vi "BuildAllFileNames.vi"(8 "Reset?":bool, 11 "Settings":T1={"Name of test"="", "Date"=timestamp(0 s since 1904-01-01), "Location"="", "Template"="", "Soundcard"="", "resolution"=32, "Sampling rate"=48000, "Ch1 Gain "=25.0, "Ch2 Gain"=10.0, "Sample time (s)"=0.3, "Pre-trigger (s)"=0.01, "Hammer Threshold"=10.0, "Positions"=12, "Taps/Position"=5, "Set Names"="", "Freq resolution"=10.0, "Hammer cutoff"=0.0, "Mic cutoff"=0.0, "Double bounce "=0.0, "Hammer Cal"=10.0, "dB Offset"=0.0, "Accel Cal"=10.0, "Vibrometer Cal"=0.0, "Mic Cal"=0.0, "Output"=2, "Voltage Cal"=1.0, "Vibrometer Port"="ASRL27::INSTR", "Range"=4, "High Pass"=2, "Bandwidth"=4, "X Range"=[], "Y Range"=[], "dB Spread"=0.0, "Trigger"=0, "Ch_1"=25, "Ch_2"=25, "flip?"=FALSE, "60Hz"=FALSE, "Time offset"=0.0, "Piezo Cal"=1.0, "Default Notes"=""} {"Ch_2" min=1 step=1; "Ch_1" min=1 max=100 step=1; "Trigger" items=["Hammer (force)", "Self-tap", "Spacebar"]; "Bandwidth" items=["1 kHz"=1, "5 kHz"=5, "10 kHz"=10, "25 kHz"=25, "50 kHz"=50, "100 kHz"=100]; "High Pass" items=["Off", "13 Hz", "104 Hz"]; "Range" items=["10 mm/s"=1, "20 mm/s"=2, "50 mm/s"=5, "100 mm/s"=10, "200 mm/s"=20, "500 mm/s"=50, "1 m/s"=100, "2 m/s"=200]; "Output" items=["Accelerometer", "Speed (from acceleration)", "Microphone", "Vibrometer", "Piezo"]; "Voltage Cal" format="%#_13g"; "Ch2 Gain" format="%#_13g"; "Ch1 Gain" format="%#_13g"; "Double bounce" min=0.0; "Mic cutoff" min=0.0 format="%#_4g"; "Hammer cutoff" min=0.0 format="%#_4g"; "Freq resolution" min=0.0; "Pre-trigger (s)" format="%#_13g"; "Date" format="%<%H:%M\n%d/%m/%y>T"; "resolution" items=["16 bit"=16, "24 bit"=24, "32 bit"=32]; "Sampling rate" items=["22050 samp/s"=22050, "44100 samp/s"=44100, "48000 samp/s"=48000]}) -> (2 "Info":cluster{i32, i32, i32}[](array[cluster]), 3 "File Names":string[](array[string]))   [LabVIEW 2022 SP3]
uses:
  PreferencesControl.ctl
panel:
  # "Hz"
  # "dB"
  # "dB"
  # "sec"
  # "sec"
  # "mV/Pa"
  # "mV/m/s2"
  # "mV/mm/s"
  # "V/N"
  # "sec"
  # "sec"
  # "mV/N"
  # "a.u."
  # "a.u."
  # "sec"
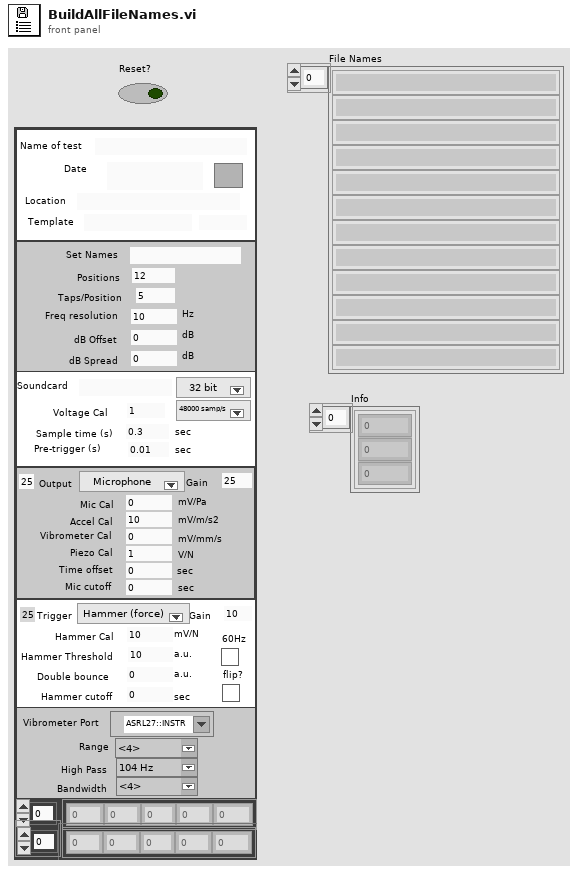
[diagram p1: front panel]
types:
  T1 = typedef "PreferencesControl.ctl" = cluster{"Name of test":string, "Date":timestamp, "Location":string, "Template":string, "Soundcard":string, "resolution":u16, "Sampling rate":u16, "Ch1 Gain ":dbl, "Ch2 Gain":dbl, "Sample time (s)":dbl, "Pre-trigger (s)":dbl, "Hammer Threshold":dbl, "Positions":i16, "Taps/Position":i16, "Set Names":string, "Freq resolution":dbl, "Hammer cutoff":dbl, "Mic cutoff":dbl, "Double bounce ":dbl, "Hammer Cal":dbl, "dB Offset":dbl, "Accel Cal":dbl, "Vibrometer Cal":dbl, "Mic Cal":dbl, "Output":u16, "Voltage Cal":dbl, "Vibrometer Port":refnum<visa-resource-name>, "Range":u16, "High Pass":u16, "Bandwidth":u16, "X Range":cluster{"Minimum":dbl, "Maximum":dbl, "Increment":dbl, "Minor Increment":dbl, "Start":dbl}[], "Y Range":cluster{"Minimum":dbl, "Maximum":dbl, "Increment":dbl, "Minor Increment":dbl, "Start":dbl}[], "dB Spread":dbl, "Trigger":u16, "Ch_1":u8, "Ch_2":u8, "flip?":bool, "60Hz":bool, "Time offset":dbl, "Piezo Cal":dbl, "Default Notes":string}
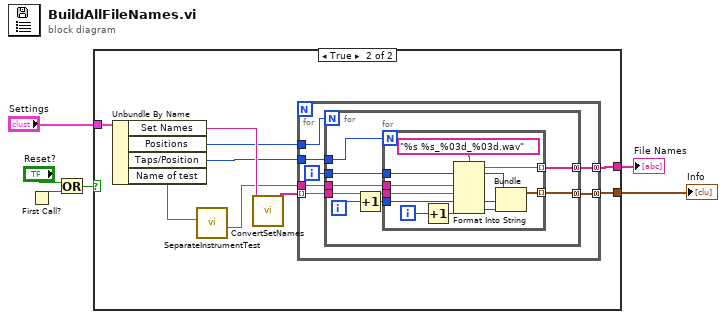
[diagram p0: block diagram]
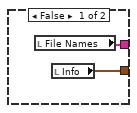
[diagram p2: hidden frame]
diagram:
  n1 = First Call?() -> (First Call?: T/F=w3:bool)
  n2 = Or(x="Reset?", y=w3) -> (x .or. y?=w1:bool)
  n3 = case shown="True" w1 {
    tunnel: "Settings" -> [_ w17]
    tunnel: [w8 w16] -> w5
    tunnel: [w7 w15] -> w4
    frame False {
      n4 = local read "File Names"() -> (w8:string[])
      n5 = local read "Info"() -> (w7:cluster{i32, i32, i32}[])
    }
    frame True {
      n6 = Unbundle By Name(w17) -> ("Set Names"=w14:string, "Positions"=w13:i16, "Taps/Position"=w12:i16, "Name of test"=w10:string)
      n7 = call "SeparateInstrumentTest.vi"("Instrument"=w10) -> ("Just test"=w9:string)  [unwired: 6 in, 4 out]
      n8 = call "ConvertSetNames.vi"("Set Names"=w14) -> ("Set Names"=w11:string[])  [unwired: 10 in]
      n9 = for {
        tunnel: w9 -> [w24]
        tunnel: w11 -> [w23] mode=indexing
        tunnel: w12 -> [w22]
        tunnel: w13 -> [w21]
        tunnel: [w20] -> w16 mode=concatenating
        tunnel: [w18] -> w15 mode=concatenating
        i -> [w19]
        n10 = for {
          N: w21 -> [_]
          tunnel: w24 -> [w32]
          tunnel: w23 -> [w31]
          tunnel: w22 -> [w30]
          tunnel: [w27] -> w20 mode=concatenating
          tunnel: w19 -> [w26]
          tunnel: [w25] -> w18 mode=concatenating
          i -> [w29]
          n11 = Increment(x=w29) -> (x+1=w28:i32)
          n12 = for {
            N: w30 -> [_]
            tunnel: w32 -> [w40]
            tunnel: w31 -> [w39]
            tunnel: w28 -> [w36]
            tunnel: [w37] -> w27 mode=indexing
            tunnel: w26 -> [w34]
            tunnel: [w33] -> w25 mode=indexing
            i -> [w38]
            n13 = Increment(x=w38) -> (x+1=w35:i32)
            n14 = Format Into String(format string="%s %s_%03d_%03d.wav", w40, w39, w36, w35) -> (resulting string=w37:string)  [unwired: 2 in, 1 out]
            n15 = Bundle(w34, w36, w35) -> (w33:cluster{i32, i32, i32})  [unwired: 1 in]
          }
        }
      }
    }
  }
  "File Names" <- w5
  "Info" <- w4
